vi "BuyProductsSabritas.vi"(8 "error in (no error)":errorcluster, 10 "Comprar":bool, 11 "Sabritas Actor in":refnum<class "Sabritas Actor.lvclass">) -> (0 "error out":errorcluster, 3 "Sabritas Actor out":refnum<class "Sabritas Actor.lvclass">)   [LabVIEW 2020, in "Sabritas Actor.lvlib" / "Sabritas Actor.lvclass"]
uses:
  Sabritas Actor.lvclass
  C:/Program Files (x86)/National Instruments/LabVIEW 2020/vi.lib/ActorFramework/Actor/Actor.lvclass
  <vilib>/ActorFramework/Actor/Actor.lvclass/Actor.ctl
  Sabritas Actor.lvclass/Sabritas Actor.ctl
  UI Actor Messages/BuyProductSabritas Msg/BuyProductSabritas Msg.lvclass/BuyProductSabritas Msg.ctl
  <vilib>/ActorFramework/Message Enqueuer/Message Enqueuer.lvclass/Message Enqueuer.ctl
  <vilib>/ActorFramework/Message Enqueuer/Enqueue.vi
  UI Actor Messages/BuyProductSabritas Msg/BuyProductSabritas Msg.lvclass
  C:/Program Files (x86)/National Instruments/LabVIEW 2020/vi.lib/ActorFramework/Message/Message.lvclass
  <vilib>/ActorFramework/Message Priority Queue/Priority Enqueue.vi
  <vilib>/ActorFramework/Actor/Actor.lvclass
panel:
  in  "Description":T1
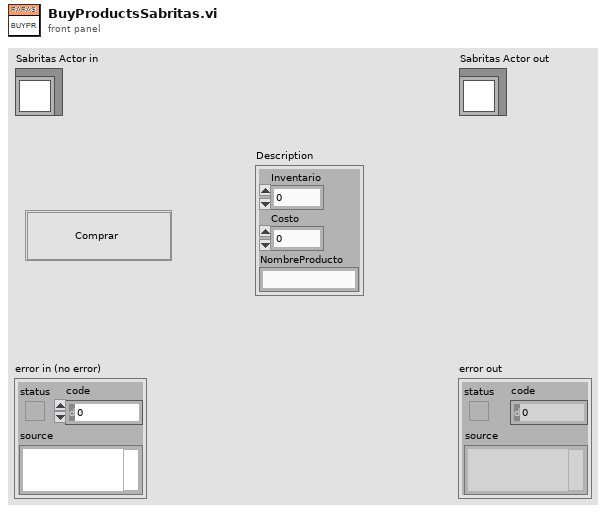
[diagram p1: front panel]
types:
  T1 = cluster{"Inventario":i32, "Costo":dbl, "NombreProducto":string}
  T2 = cluster{"Data[0]":string, "Data[1]":string, "Data[2]":string, "Data[3]":string, "Data[4]":string, "Data[5]":string, "Data[6]":string, "Data[7]":string, "Data[8]":string}
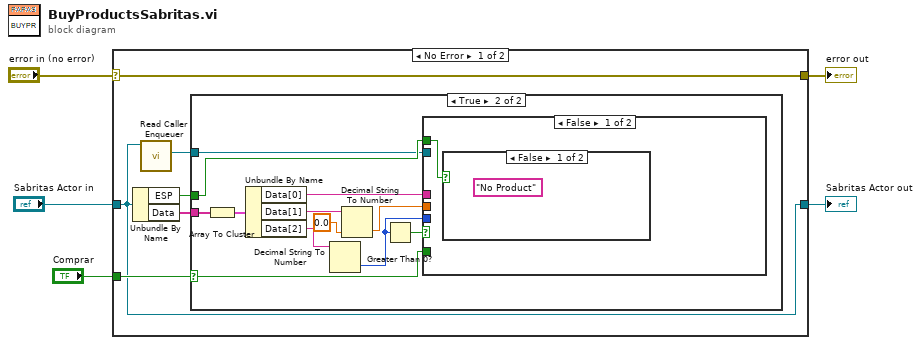
[diagram p0: block diagram]
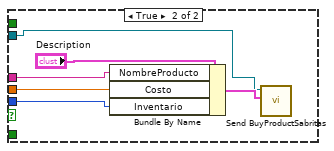
[diagram p4: hidden frame]
diagram:
  n1 = case shown="No Error" "error in (no error)" {
    selector: "error in (no error)" -> [w11 w32]
    tunnel: [w11 w32] -> w4
    tunnel: [w6 w31] -> w2
    tunnel: "Sabritas Actor in" -> [w6 w31]
    tunnel: "Comprar" -> [w7 _]
    frame No Error {
      n2 = Unbundle By Name(w6) -> ("ESP"=w9:bool, "Data"=w10:string[])
      n3 = call <vilib>:"Read Caller Enqueuer.vi"("Actor"=w6) -> ("Caller Enqueuer"=w8:refnum<class "Message Enqueuer.lvclass">)  [unwired: 10 in]
      n4 = case shown="True" w7 {
        selector: w7 -> [_ w15]
        tunnel: w10 -> [_ w23]
        tunnel: w9 -> [_ w20]
        tunnel: w8 -> [_ w14]
        frame False {
        }
        frame True {
          n5 = Array To Cluster(array=w23) -> (cluster=w22:T2)
          n6 = Unbundle By Name(w22) -> ("Data[0]"=w17:string, "Data[1]"=w13:string, "Data[2]"=w12:string)
          n7 = Decimal String To Number(string=w12) -> (number=w16:i32)  [unwired: 2 in, 1 out]
          n8 = Decimal String To Number(string=w13, default (0L)=0.0) -> (number=w18:dbl)  [unwired: 1 in, 1 out]
          n9 = Greater Than 0?(x=w16) -> (x > 0?=w19:bool)
          n10 = case shown="False" w19 {
            tunnel: w18 -> [_ w29]
            tunnel: w20 -> [w24 _]
            tunnel: w17 -> [_ w27]
            tunnel: w16 -> [_ w28]
            tunnel: w15 -> [_ _]
            tunnel: w14 -> [_ w25]
            frame False {
              n11 = case shown="False" w24 {
                frame False {
                  (unwired) "No Product"
                }
                frame True {
                }
              }
            }
            frame True {
              n12 = Bundle By Name(cluster="Description", "NombreProducto"=w27, "Costo"=w29, "Inventario"=w28) -> (w26:T1)
              n13 = call "Send BuyProductSabritas.vi"("Description"=w26, "Message Enqueuer"=w25) -> ()  [unwired: 8 in, 2 out]
            }
          }
        }
      }
    }
    frame Error {
    }
  }
  "error out" <- w4
  "Sabritas Actor out" <- w2
